vi "div3jk_v8.vi"() -> ()   [LabVIEW 2014]
panel:
  in  "K 2":T1(ring)=enum."1"
  in  "K 1":T1(ring)=enum."1"
  in  "J 2":T1(ring)
  in  "J 1":T1(ring)=enum."Q2 barra"
  in  "Stato iniziale":enum8{"0 0", "0 1", "1 0", "1 1"}(ring)
  out "A 2":bool[][](array[boolean])=[[FALSE, FALSE], [TRUE, FALSE], [FALSE, TRUE], [FALSE, FALSE], [TRUE, FALSE], [FALSE, TRUE], [FALSE, FALSE], [TRUE, FALSE], [FALSE, TRUE], [FALSE, FALSE], [TRUE, FALSE], [FALSE, TRUE], [FALSE, FALSE], [TRUE, FALSE], [FALSE, TRUE], [FALSE, FALSE], [TRUE, FALSE], [FALSE, TRUE], [FALSE, FALSE], [FALSE, FALSE], [FALSE, FALSE], [FALSE, FALSE], [FALSE, FALSE], [FALSE, FALSE], [FALSE, FALSE], [FALSE, FALSE], [FALSE, FALSE], [FALSE, FALSE], [FALSE, FALSE], [FALSE, FALSE], [FALSE, FALSE], [FALSE, FALSE], [FALSE, FALSE], [FALSE, FALSE], [FALSE, FALSE], [FALSE, FALSE], [FALSE, FALSE], [FALSE, FALSE], [FALSE, FALSE], [FALSE, FALSE]]
  out "B":bool=TRUE
  out "A":bool
  in  "impulsi":u32=17
  in  "CLK":bool
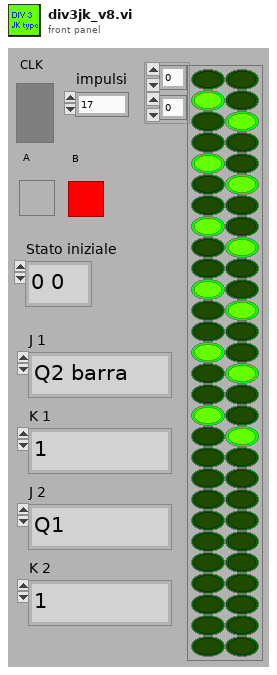
[diagram p1: front panel]
types:
  T1 = enum8{"Q1", "Q1 barra", "Q2 ", "Q2 barra", "0", "1"}
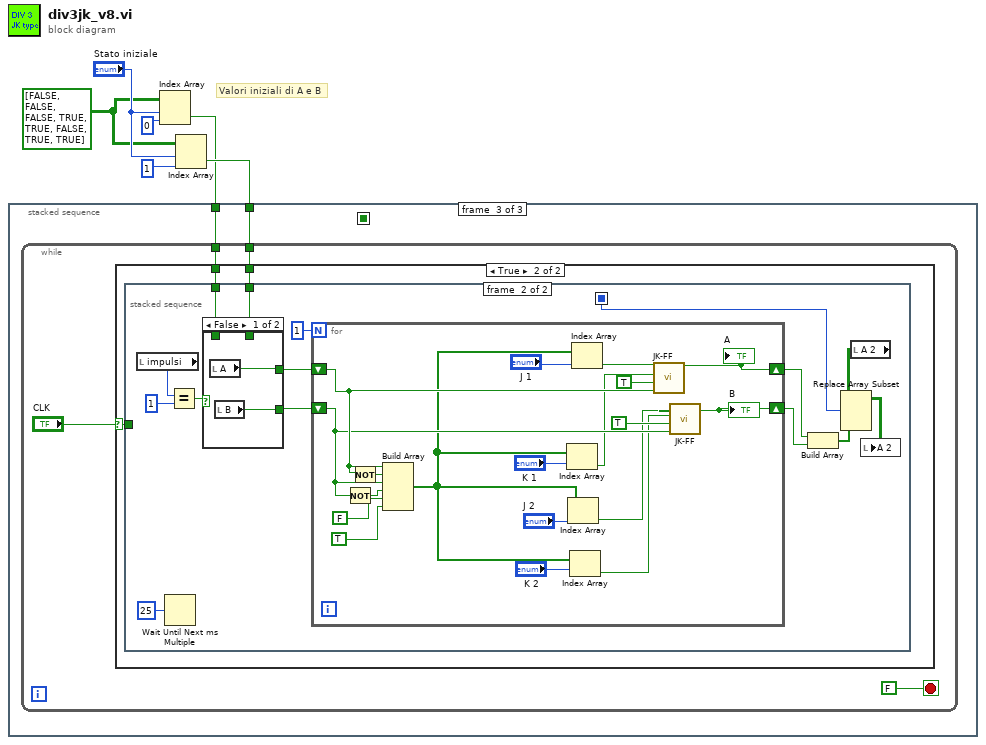
[diagram p0: block diagram]
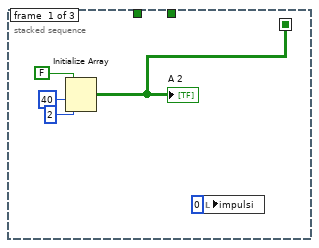
[diagram p2: hidden frame]
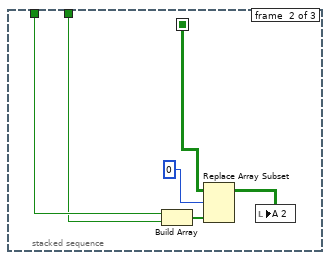
[diagram p3: hidden frame]
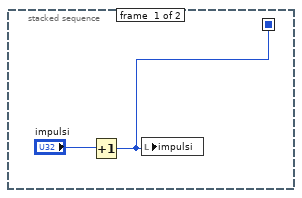
[diagram p5: hidden frame]
diagram:
  w1 = bool[][] [[FALSE, FALSE], [FALSE, TRUE], [TRUE, FALSE], [TRUE, TRUE]]
  # "Valori iniziali di A e B"
  n1 = Index Array(array=w1, index (row)="Stato iniziale", index (col)=0 ("disabled index (col)")) -> (element=w2:bool)
  n2 = Index Array(array=w1, index (row)="Stato iniziale", index (col)=1 ("length")) -> (element=w3:bool)
  n3 = stacked-sequence {
    seq-local: [w7 _ _] -> [_ w13 _]
    tunnel: w2 -> [_ w15 w19]
    tunnel: w3 -> [_ w14 w18]
    frame #0 {
      n4 = Initialize Array(FALSE ("Boolean"), 40 ("dimension size"), 2 ("dimension size")) -> (w7:bool[][])
      "A 2" <- w7
      n5 = local write "impulsi"(u32 0 ("impulsi")) -> ()
    }
    frame #1 {
      n6 = Build Array(w15, w14) -> (w16:bool[])
      n7 = Replace Array Subset(array=w13, new element=w16, index (row)=0) -> (w12:bool[][])  [unwired: 1 in]
      n8 = local write "A 2"(w12) -> ()
    }
    frame #2 {
      n9 = while {
        tunnel: w19 -> [w21]
        tunnel: w18 -> [w20]
        stop <- FALSE stop-if-true
        n10 = case shown="True" "CLK" {
          selector: "CLK" -> [_ w26]
          tunnel: w21 -> [_ w25]
          tunnel: w20 -> [_ w24]
          frame False {
          }
          frame True {
            n11 = stacked-sequence {
              seq-local: [w27 _] -> [_ w31]
              tunnel: w26 -> [_ _]
              tunnel: w25 -> [_ w36]
              tunnel: w24 -> [_ w35]
              frame #0 {
                n12 = Increment(x="impulsi") -> (x+1=w27:u32)
                n13 = local write "impulsi"(w27) -> ()
              }
              frame #1 {
                n14 = local read "impulsi"() -> (w42:u32)
                n15 = Wait Until Next ms Multiple(millisecond multiple=u32 25) -> ()  [unwired: 1 out]
                n16 = Equal?(x=w42, y=u32 1) -> (x = y?=w37:bool)
                n17 = case shown="False" w37 {
                  tunnel: [w45 w46] -> w40
                  tunnel: [w44 w47] -> w38
                  tunnel: w36 -> [_ w47]
                  tunnel: w35 -> [_ w46]
                  frame False {
                    n18 = local read "A"() -> (w44:bool)
                    n19 = local read "B"() -> (w45:bool)
                  }
                  frame True {
                  }
                }
                n20 = for {
                  N: 1 -> [_]
                  shift-right: [w64] -> w32
                  shift-left: w40 -> [w60]
                  shift-right: [w63] -> w33
                  shift-left: w38 -> [w62]
                  n21 = Not(x=w60) -> (.not. x?=w59:bool)
                  n22 = Not(x=w62) -> (.not. x?=w61:bool)
                  n23 = Build Array(w62, w61, w60, w59, FALSE, TRUE) -> (w54:bool[])
                  n24 = Index Array(array=w54, index="K 1") -> (element=w56:bool)
                  n25 = Index Array(array=w54, index="J 2") -> (element=w55:bool)
                  n26 = Index Array(array=w54, index="K 2") -> (element=w53:bool)
                  n27 = Index Array(array=w54, index="J 1") -> (element=w57:bool)
                  n28 = call "JK-FF.vi"("Qprev"=w62, "CLK"=TRUE, "K"=w56, "J"=w57) -> ("Q"=w63:bool)  [unwired: 1 out]
                  "A" <- w63
                  n29 = call "JK-FF.vi"("Qprev"=w60, "CLK"=TRUE, "K"=w53, "J"=w55) -> ("Q"=w64:bool)  [unwired: 1 out]
                  "B" <- w64
                }
                n30 = Build Array(w33, w32) -> (w34:bool[])
                n31 = local read "A 2"() -> (w30:bool[][])
                n32 = Replace Array Subset(array=w30, new element=w34, index (row)=w31) -> (w29:bool[][])  [unwired: 1 in]
                n33 = local write "A 2"(w29) -> ()
              }
            }
          }
        }
      }
    }
  }
